vi "16路数字量输入判断.vi"(8 "反馈值":bool[](array[boolean]), 9 "输入值":enum16{"0", "1"}[](array[ring]), 11 "是否选择":bool[](array[boolean])) -> (0 "合格":bool, 2 "结果":cluster{u32, u32}[][](array[cluster])=[[{6618880, 6618880}]], 3 "反馈值字符串":string[](array[string]))   [LabVIEW 2010]
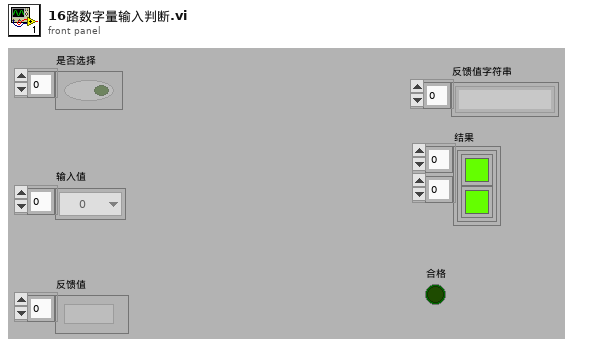
[diagram p1: front panel]
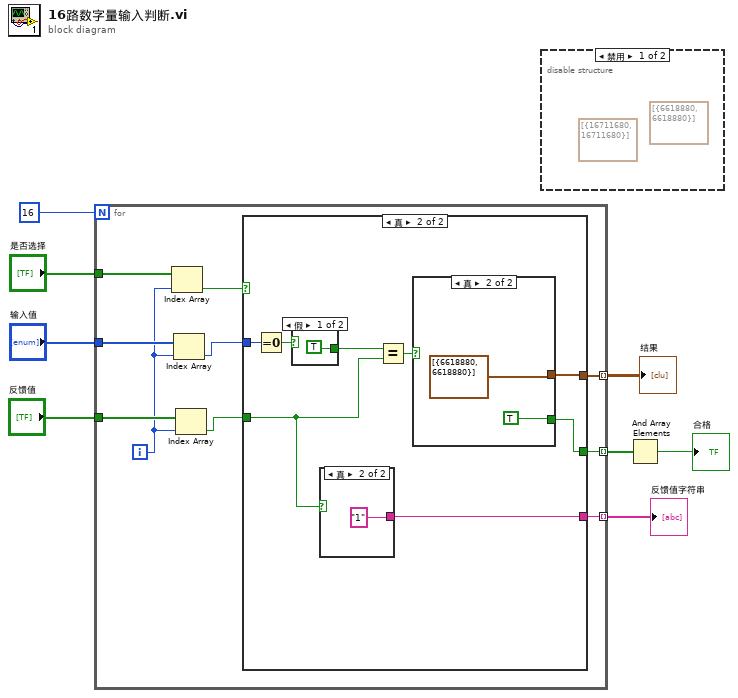
[diagram p0: block diagram]
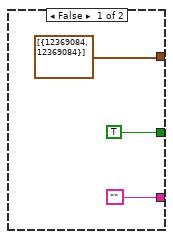
[diagram p3: hidden frame]
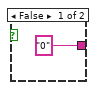
[diagram p4: hidden frame]
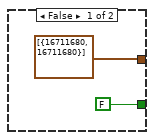
[diagram p5: hidden frame]
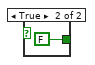
[diagram p6: hidden frame]
diagram:
  n1 = for {
    N: 16 -> [_]
    tunnel: "是否选择" -> [w15]
    tunnel: "输入值" -> [w14]
    tunnel: "反馈值" -> [w13]
    tunnel: [w18] -> w4 mode=indexing
    tunnel: [w17] -> w3 mode=indexing
    tunnel: [w16] -> w1 mode=indexing
    i -> [w12]
    n2 = Index Array(array=w15, index=w12) -> (element=w11:bool)
    n3 = Index Array(array=w14, index=w12) -> (element=w10:enum16{"0", "1"})
    n4 = Index Array(array=w13, index=w12) -> (element=w9:bool)
    n5 = case shown="真" w11 {
      tunnel: w10 -> [_ w29]
      tunnel: w9 -> [_ w23]
      tunnel: [cluster{u32, u32}[] [{12369084, 12369084}] w26] -> w18
      tunnel: [TRUE w24] -> w17
      tunnel: ["" w22] -> w16
      frame False {
      }
      frame True {
        n6 = Equal To 0?(x=w29) -> (x = 0?=w25:bool)
        n7 = case shown="假" w25 {
          tunnel: [TRUE FALSE] -> w27
          frame False {
          }
          frame True {
          }
        }
        n8 = case shown="真" w23 {
          tunnel: ["0" "1"] -> w22
          frame False {
          }
          frame True {
          }
        }
        n9 = Equal?(x=w27, y=w23) -> (x = y?=w28:bool)
        n10 = case shown="真" w28 {
          tunnel: [cluster{u32, u32}[] [{16711680, 16711680}] cluster{u32, u32}[] [{6618880, 6618880}]] -> w26
          tunnel: [FALSE TRUE] -> w24
          frame False {
          }
          frame True {
          }
        }
      }
    }
  }
  "结果" <- w4
  "反馈值字符串" <- w1
  n11 = disable-structure shown="禁用" {
    frame Disabled {
      (unwired) cluster{u32, u32}[] [{6618880, 6618880}]
      (unwired) cluster{u32, u32}[] [{16711680, 16711680}]
    }
    frame Enabled {
    }
  }
  n12 = And Array Elements(Boolean array=w3) -> (logical AND=→"合格":bool)
